vi "secondaryfilter_GUI.vi"(4 "error in (no error)":errorcluster, 7 "connection ID":refnum<k5>) -> (0 "error out":errorcluster)   [LabVIEW 2015]
doc: "Use this template to build a PDA VI for Pocket PC 2002 devices or emulators."
panel:
  out "Filter Names":string
  in  "Filter #":i32(ring) items=["0", "1", "2", "3", "4", "5"]
  in  "Cancel":bool
  in  "OK":bool
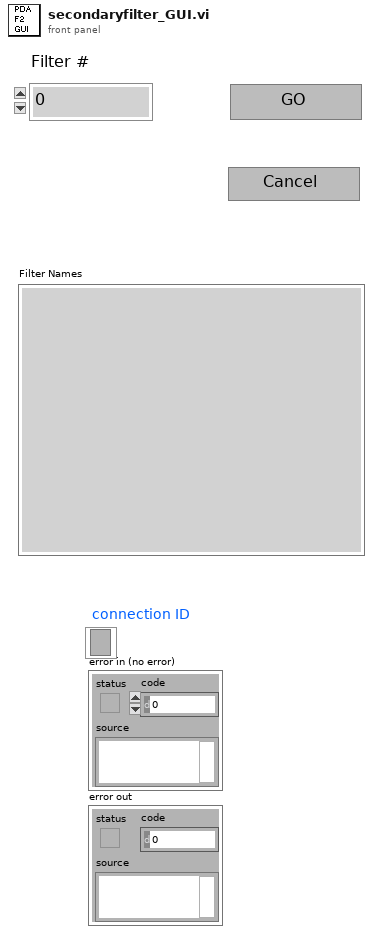
[diagram p1: front panel]
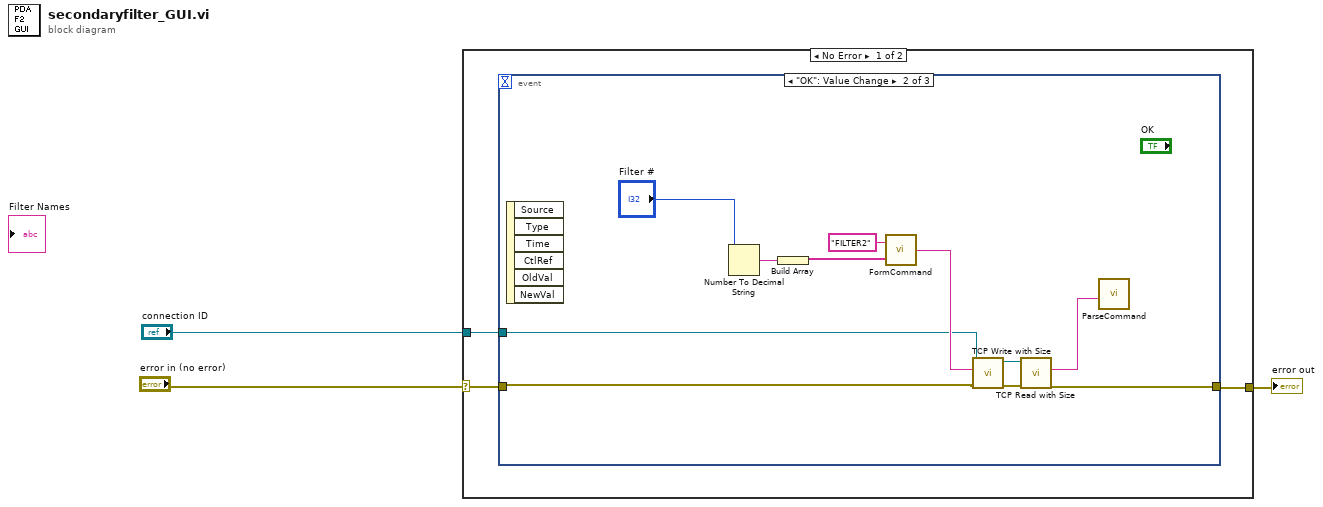
[diagram p0: block diagram]
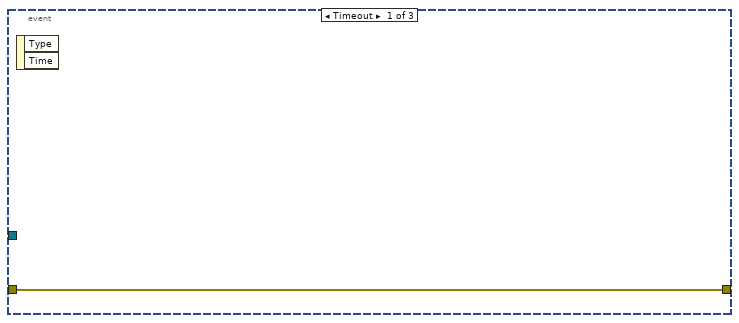
[diagram p2: hidden frame]
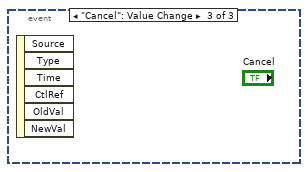
[diagram p3: hidden frame]
diagram:
  n1 = case shown="No Error" "error in (no error)" {
    selector: "error in (no error)" -> [w6 w19]
    tunnel: [w5 w19] -> w3
    tunnel: "connection ID" -> [w4 _]
    frame No Error {
      n2 = event shown="[1] \"OK\": Value Change" {
        selector: _ -> [_ _ _]
        dyn-events: _ -> [_ _ _]
        timeout: _ -> [_ _ _]
        tunnel: w6 -> [w7 w11 _]
        tunnel: [w7 w8 _] -> w5
        tunnel: w4 -> [_ w10 _]
        event Timeout {
          n3 = event-data() -> ()  [unwired: 1 in, 2 out]
        }
        event "OK": Value Change {
          n4 = event-data() -> ()  [unwired: 1 in, 6 out]
          n5 = Number To Decimal String(number="Filter #") -> (decimal integer string=w17:string)  [unwired: 1 in]
          n6 = Build Array(w17) -> (w16:string[])
          n7 = call "FormCommand.vi"("Parameters"=w16, "Command"="FILTER2") -> ("Command string"=w15:string)
          n8 = call "TCP Write with Size.vi"("error in (no error)"=w11, "data in"=w15, "connection ID"=w10) -> ("error out"=w9:errorcluster, "connection ID out"=w14:refnum<k5>)  [unwired: 6 in, 1 out]
          n9 = call "TCP Read with Size.vi"("error in (no error)"=w9, "connection ID"=w14) -> ("error out"=w8:errorcluster, "data out"=w13:string)  [unwired: 7 in, 1 out]
          n10 = call "ParseCommand.vi"("Command string"=w13) -> ()  [unwired: 2 out]
        }
        event "Cancel": Value Change {
          n11 = event-data() -> ()  [unwired: 1 in, 6 out]
        }
      }
    }
    frame Error {
    }
  }
  "error out" <- w3
